vi "ZAlign_Remove_empty_ctrls.vi"(2 "TermBnds[]":T1[](array[typedef]), 3 "Controls in":refnum<vi>[](array[refnum])) -> (0 "Control locations":T1[](array[typedef]), 1 "Controls out":refnum<vi>[](array[refnum]))   [LabVIEW 2014, in "ZAlign.lvlib"]
doc: "ZAlign.lvlib:ZAlign_Remove_empty_ctrls.vi\n----------------------------------------------\nRemove empty Controls\n\nInputs:\n---------------------\n- TermBnds[] : 1DArrayOfCluster; \n- Controls in : 1DArrayOfRefnum; \n\nOutputs:\n---------------------\n- Control locations : 1DArrayOfCluster; \n- Controls out : 1DArrayOfRefnum; \n\n----------------------------------------------\n16/03/2015\nZühlke Engineering AG\nCH-8952 Schlieren\nwww.zuehlke.com"
uses:
  ZAlign.lvlib
  <vilib>/Utility/miscctls.llb/LVRectTypeDef.ctl
panel:
  # "Connector Pane"
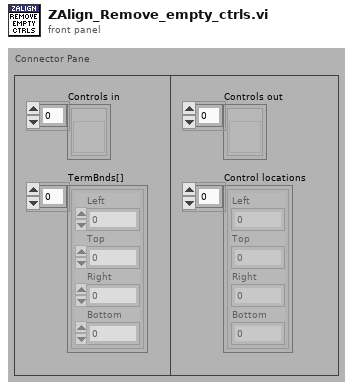
[diagram p1: front panel]
types:
  T1 = typedef "LVRectTypeDef.ctl" = cluster{"Left":i16, "Top":i16, "Right":i16, "Bottom":i16}
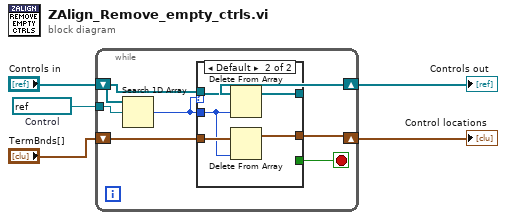
[diagram p0: block diagram]
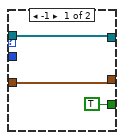
[diagram p2: hidden frame]
diagram:
  w4 = refnum<vi> refnum  # Control
  n1 = while {
    tunnel: w4 -> [w6]
    shift-right: [w11] -> w5
    shift-left: "Controls in" -> [w12]
    shift-right: [w7] -> w1
    shift-left: "TermBnds[]" -> [w8]
    stop <- w9 stop-if-true
    n2 = Search 1D Array(1D array=w12, element=w6) -> (index of element=w10:i32)  [unwired: 1 in]
    n3 = case shown="Default" w10 {
      tunnel: w10 -> [_ w16]
      tunnel: w12 -> [w15 w20]
      tunnel: [w15 w19] -> w11
      tunnel: [TRUE _] -> w9
      tunnel: w8 -> [w13 w18]
      tunnel: [w13 w17] -> w7
      frame -1 {
      }
      frame Default {
        n4 = Delete From Array(array=w20, index=w16) -> (array with subset deleted=w19:refnum<vi>[])  [unwired: 1 in, 1 out]
        n5 = Delete From Array(array=w18, index=w16) -> (array with subset deleted=w17:T1[])  [unwired: 1 in, 1 out]
      }
    }
  }
  "Control locations" <- w1
  "Controls out" <- w5
